vi "LVJSON to Variant.vi"(8 "error in (no error)":errorcluster, 10 "Variant Type":variant, 11 "Root Element in":T1) -> (0 "error out":errorcluster, 2 "Key":string, 3 "Variant out":variant)   [LabVIEW 2019, in "labview_json.lvlib"]
uses:
  labview_json.lvlib
  Element.ctl
  Element Type.ctl
  <vilib>/Utility/error.llb/Error Cluster From Error Code.vi
  <vilib>/ErrorRing/Error Ring.xnode
  <vilib>/Utility/Data Type/NI_Data Type.lvlib
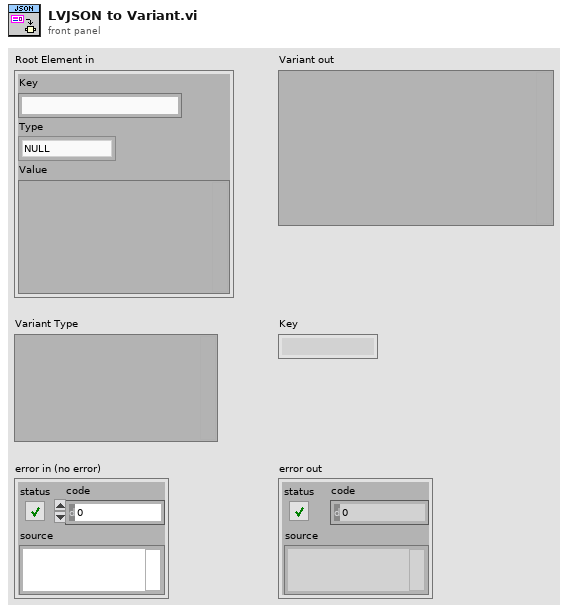
[diagram p1: front panel]
types:
  T1 = typedef "labview_json.lvlib/Element.ctl" = cluster{"Key":string, "Type":T2, "Value":variant}
  T2 = typedef "labview_json.lvlib/Element Type.ctl" = enum8{"NULL", "OBJECT", "ARRAY", "BOOL", "INT", "UINT", "FLOAT", "STRING"}
  T3 = typedef "NI_Data Type.lvlib/Data Type.ctl" = enum8{"Invalid Type", "Void", "I8", "I16", "I32", "I64", "U8", "U16", "U32", "U64", "Single Float", "Double Float", "Extended Float", "Single Complex", "Double Complex", "Extended Complex", "Enum U8", "Enum U16", "Enum U32", "Enum U64", "Single Float With Unit", "Double Float With Unit", "Extended Float With Unit", "Single Complex with Unit", "Double Complex with Unit", "Extended Complex with Unit", "Boolean", "String", "Path", "Picture", "Tag", "Array", "Cluster", "Variant", "LV Variant", "Waveform", "Timestamp", "Digital Waveform", "Digital Data", "ExpressData", "Refnum", "External Data", "VI", "Poly VI", "LabVIEW Class Instance", "Fixed Point", "Set Collection", "Map Collection"}
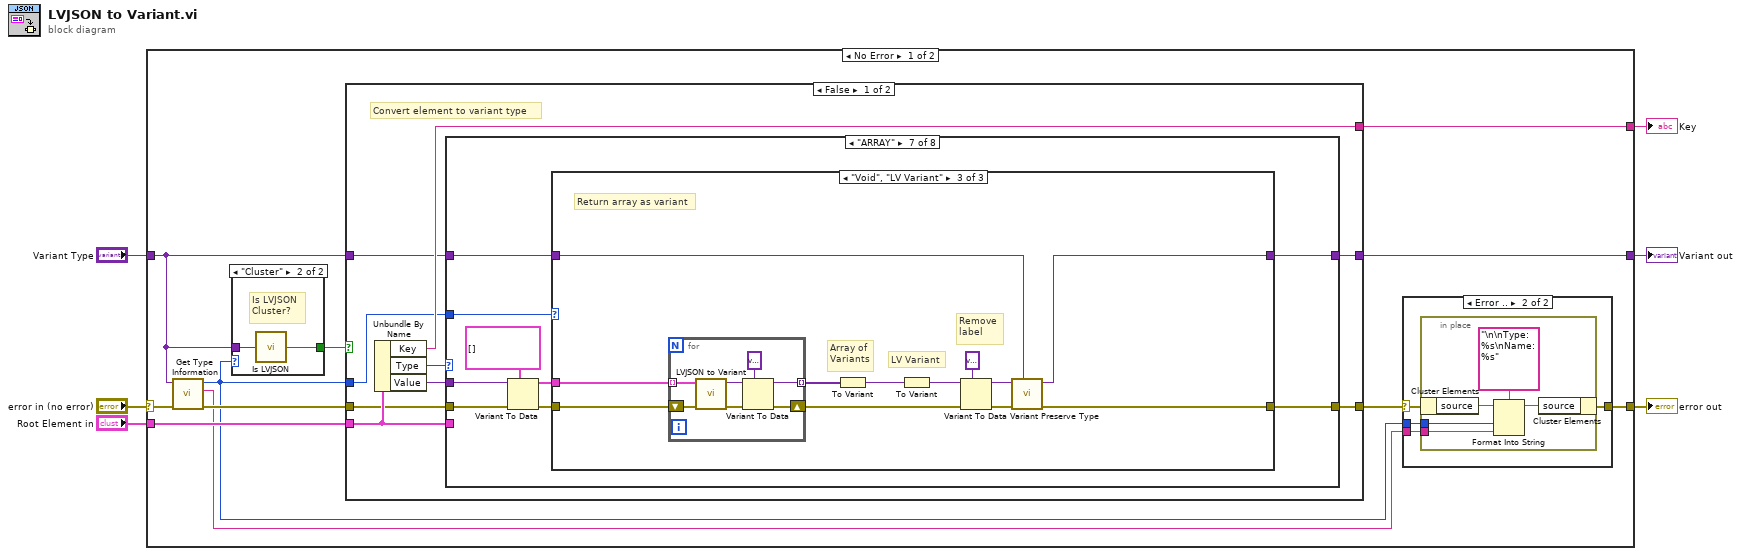
[diagram p0: block diagram]
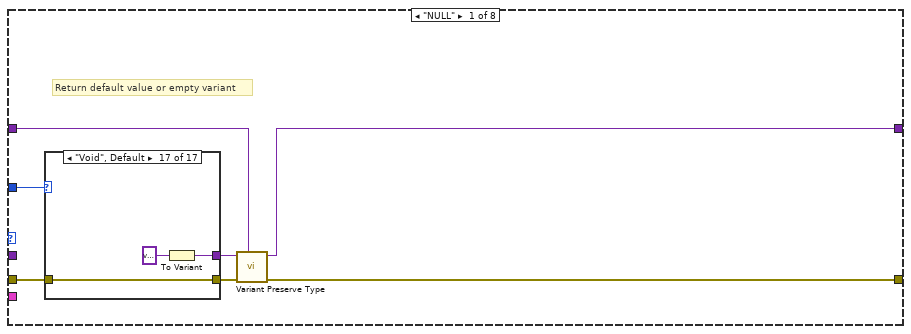
[diagram p2: hidden frame]
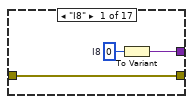
[diagram p3: hidden frame]
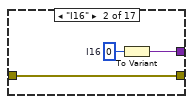
[diagram p4: hidden frame]
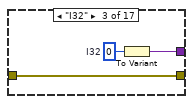
[diagram p5: hidden frame]
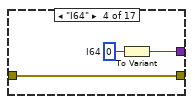
[diagram p6: hidden frame]
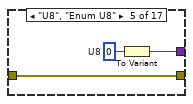
[diagram p7: hidden frame]
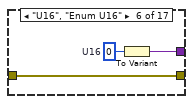
[diagram p8: hidden frame]
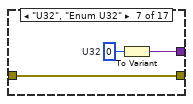
[diagram p9: hidden frame]
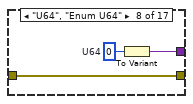
[diagram p10: hidden frame]
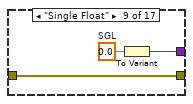
[diagram p11: hidden frame]
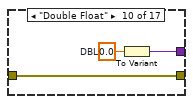
[diagram p12: hidden frame]
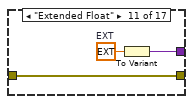
[diagram p13: hidden frame]
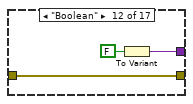
[diagram p14: hidden frame]
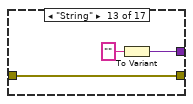
[diagram p15: hidden frame]
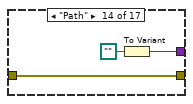
[diagram p16: hidden frame]
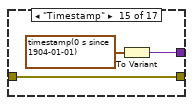
[diagram p17: hidden frame]
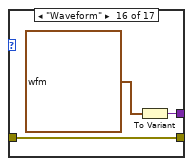
[diagram p18: hidden frame]
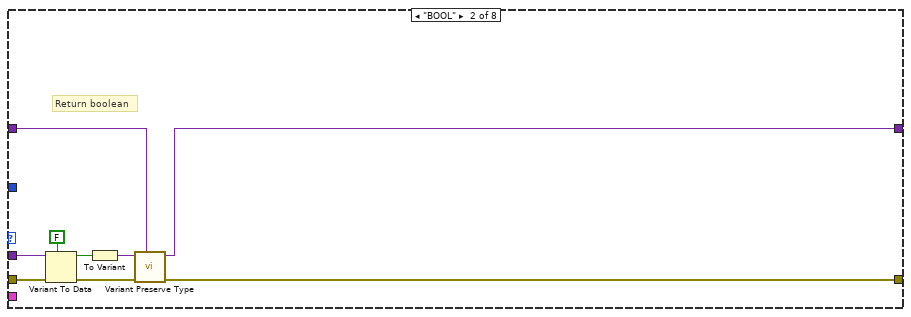
[diagram p19: hidden frame]
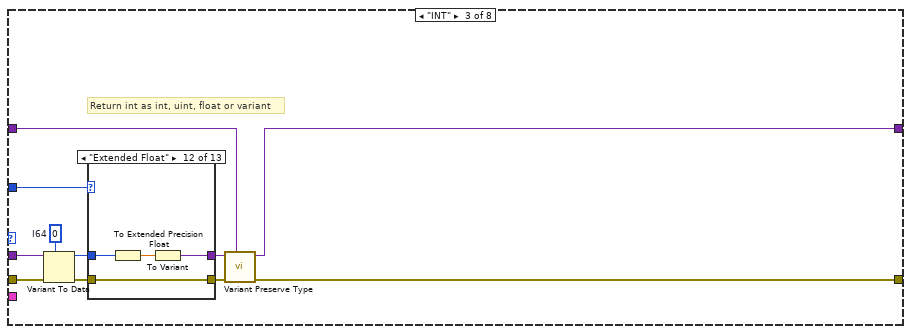
[diagram p20: hidden frame]
diagram:
  n1 = case shown="No Error" "error in (no error)" {
    selector: "error in (no error)" -> [w14 w587]
    tunnel: "Root Element in" -> [w15 _]
    tunnel: [w17 w587] -> w6
    tunnel: "Variant Type" -> [w13 w586]
    tunnel: [w16 _] -> w2
    tunnel: [w12 w586] -> w1
    frame No Error {
      n2 = call <vilib>:"Get Type Information.vi"("error in (no error)"=w14, "variant"=w13) -> ("error out"=w11:errorcluster, "name"=w9:string, "type"=w8:T3)  [unwired: 5 in, 2 out]
      n3 = case shown="\"Cluster\"" w8 {
        tunnel: w13 -> [_ w575]
        tunnel: [_ w574] -> w7
        frame Default {
        }
        frame "Cluster" {
          # "Is LVJSON\nCluster?"
          n4 = call "Is LVJSON.vi"("Variant"=w575) -> ("Is LVJSON?"=w574:bool)
        }
      }
      n5 = case shown="False" w7 {
        tunnel: [w26 w571] -> w16
        tunnel: w15 -> [w25 w572]
        tunnel: w13 -> [w24 _]
        tunnel: [w23 w573] -> w12
        tunnel: w11 -> [w22 w570]
        tunnel: [w21 w570] -> w10
        tunnel: w8 -> [w18 _]
        frame False {
          # "Convert element to variant type"
          n6 = Unbundle By Name(w25) -> ("Key"=w26:string, "Type"=w20:T2, "Value"=w19:variant)
          n7 = case shown="\"ARRAY\"" w20 {
            tunnel: [w31 w93 w104 w166 w228 w290 w343 w434] -> w23
            tunnel: w22 -> [w33 w88 w98 w160 w222 w285 w349 w440]
            tunnel: w24 -> [w29 w91 w102 w164 w226 w282 w344 w435]
            tunnel: w25 -> [_ _ _ _ _ _ _ w432]
            tunnel: w19 -> [_ w87 w97 w159 w221 w284 w348 w439]
            tunnel: w18 -> [w32 _ w96 w156 w220 w283 w347 w438]
            tunnel: [w30 w92 w103 w165 w227 w289 w342 w433] -> w21
            frame "NULL" {
              # "Return default value or empty variant"
              n8 = case shown="\"Void\", Default" w32 {
                tunnel: [w36 w39 w42 w45 w48 w51 w54 w57 w60 w63 w66 w69 w72 w75 w78 w81 w84] -> w28
                tunnel: w33 -> [w36 w39 w42 w45 w48 w51 w54 w57 w60 w63 w66 w69 w72 w75 w78 w81 w84]
                tunnel: [w35 w38 w41 w44 w47 w50 w53 w56 w59 w62 w65 w68 w71 w74 w77 w80 w83] -> w27
                frame "I8" {
                  w34 = i8 0  # I8
                  n9 = To Variant(anything=w34) -> (Variant=w35:variant)
                }
                frame "I16" {
                  w37 = i16 0  # I16
                  n10 = To Variant(anything=w37) -> (Variant=w38:variant)
                }
                frame "I32" {
                  w40 = 0  # I32
                  n11 = To Variant(anything=w40) -> (Variant=w41:variant)
                }
                frame "I64" {
                  w43 = i64 0  # I64
                  n12 = To Variant(anything=w43) -> (Variant=w44:variant)
                }
                frame "U8", "Enum U8" {
                  w46 = u8 0  # U8
                  n13 = To Variant(anything=w46) -> (Variant=w47:variant)
                }
                frame "U16", "Enum U16" {
                  w49 = u16 0  # U16
                  n14 = To Variant(anything=w49) -> (Variant=w50:variant)
                }
                frame "U32", "Enum U32" {
                  w52 = u32 0  # U32
                  n15 = To Variant(anything=w52) -> (Variant=w53:variant)
                }
                frame "U64", "Enum U64" {
                  w55 = u64 0  # U64
                  n16 = To Variant(anything=w55) -> (Variant=w56:variant)
                }
                frame "Single Float" {
                  w58 = sgl 0.0  # SGL
                  n17 = To Variant(anything=w58) -> (Variant=w59:variant)
                }
                frame "Double Float" {
                  w61 = 0.0  # DBL
                  n18 = To Variant(anything=w61) -> (Variant=w62:variant)
                }
                frame "Extended Float" {
                  w64 = ext 0.0  # EXT
                  n19 = To Variant(anything=w64) -> (Variant=w65:variant)
                }
                frame "Boolean" {
                  n20 = To Variant(anything=FALSE) -> (Variant=w68:variant)
                }
                frame "String" {
                  n21 = To Variant(anything="") -> (Variant=w71:variant)
                }
                frame "Path" {
                  n22 = To Variant(anything=path "" ("Not A Path Constant")) -> (Variant=w74:variant)
                }
                frame "Timestamp" {
                  n23 = To Variant(anything=timestamp(0 s since 1904-01-01)) -> (Variant=w77:variant)
                }
                frame "Waveform" {
                  n24 = To Variant(anything=waveform(dbl) {"t0"=timestamp(0 s since 1904-01-01), "dt"=1.0, "Y"=[]} ("Waveform")) -> (Variant=w80:variant)
                }
                frame "Void", Default {
                  n25 = To Variant(anything=variant) -> (Variant=w83:variant)
                }
              }
              n26 = call "Variant Preserve Type.vi"("Variant Type"=w29, "error in (no error)"=w28, "Variant in"=w27) -> ("error out"=w30:errorcluster, "Variant out"=w31:variant)  [unwired: 7 in]
            }
            frame "BOOL" {
              # "Return boolean"
              n27 = Variant To Data(error in=w88, type=FALSE, Variant=w87) -> (data=w90:bool, error out=w86:errorcluster)
              n28 = To Variant(anything=w90) -> (Variant=w85:variant)
              n29 = call "Variant Preserve Type.vi"("Variant Type"=w91, "error in (no error)"=w86, "Variant in"=w85) -> ("error out"=w92:errorcluster, "Variant out"=w93:variant)  [unwired: 7 in]
            }
            frame "INT" {
              w101 = i64 0  # I64
              # "Return int as int, uint, float or variant"
              n30 = Variant To Data(error in=w98, type=w101, Variant=w97) -> (data=w99:i64, error out=w100:errorcluster)
              n31 = case shown="\"Extended Float\"" w96 {
                tunnel: [w107 w110 w114 w118 w122 w126 w130 w134 w138 w142 w146 w150 w155] -> w95
                tunnel: w100 -> [w107 w110 w114 w118 w122 w126 w130 w134 w138 w142 w146 w150 w155]
                tunnel: [w105 w108 w112 w116 w120 w124 w128 w132 w136 w140 w144 w148 w153] -> w94
                tunnel: w99 -> [w106 w111 w115 w119 w123 w127 w131 w135 w139 w143 w147 w151 w154]
                frame "Void", Default {
                  n32 = To Variant(anything=w106) -> (Variant=w105:variant)
                }
                frame "I8" {
                  n33 = To Byte Integer(number=w111) -> (8bit integer=w109:i8)
                  n34 = To Variant(anything=w109) -> (Variant=w108:variant)
                }
                frame "I16" {
                  n35 = To Word Integer(number=w115) -> (16bit integer=w113:i16)
                  n36 = To Variant(anything=w113) -> (Variant=w112:variant)
                }
                frame "I32" {
                  n37 = To Long Integer(number=w119) -> (32bit integer=w117:i32)
                  n38 = To Variant(anything=w117) -> (Variant=w116:variant)
                }
                frame "I64" {
                  n39 = To Quad Integer(1:w123) -> (0:w121:i64)
                  n40 = To Variant(anything=w121) -> (Variant=w120:variant)
                }
                frame "U8", "Enum U8" {
                  n41 = To Unsigned Byte Integer(number=w127) -> (unsigned 8bit integer=w125:u8)
                  n42 = To Variant(anything=w125) -> (Variant=w124:variant)
                }
                frame "U16", "Enum U16" {
                  n43 = To Unsigned Word Integer(number=w131) -> (unsigned 16bit integer=w129:u16)
                  n44 = To Variant(anything=w129) -> (Variant=w128:variant)
                }
                frame "U32", "Enum U32" {
                  n45 = To Unsigned Long Integer(number=w135) -> (unsigned 32bit integer=w133:u32)
                  n46 = To Variant(anything=w133) -> (Variant=w132:variant)
                }
                frame "U64", "Enum U64" {
                  n47 = To Unsigned Quad Integer(1:w139) -> (0:w137:u64)
                  n48 = To Variant(anything=w137) -> (Variant=w136:variant)
                }
                frame "Single Float" {
                  n49 = To Single Precision Float(number=w143) -> (single precision float=w141:sgl)
                  n50 = To Variant(anything=w141) -> (Variant=w140:variant)
                }
                frame "Double Float" {
                  n51 = To Double Precision Float(number=w147) -> (double precision float=w145:dbl)
                  n52 = To Variant(anything=w145) -> (Variant=w144:variant)
                }
                frame "Extended Float" {
                  n53 = To Extended Precision Float(1:w151) -> (0:w149:ext)
                  n54 = To Variant(anything=w149) -> (Variant=w148:variant)
                }
                frame "LV Variant" {
                  n55 = To Variant(anything=w154) -> (Variant=w152:variant)
                  n56 = To Variant(anything=w152) -> (Variant=w153:variant)
                }
              }
              n57 = call "Variant Preserve Type.vi"("Variant Type"=w102, "error in (no error)"=w95, "Variant in"=w94) -> ("error out"=w103:errorcluster, "Variant out"=w104:variant)  [unwired: 7 in]
            }
            frame "UINT" {
              w163 = u64 0  # U64
              # "Return uint as int, uint, float, enum or variant"
              n58 = Variant To Data(error in=w160, type=w163, Variant=w159) -> (data=w161:u64, error out=w162:errorcluster)
              n59 = case shown="\"Extended Float\"" w156 {
                tunnel: [w169 w172 w176 w180 w184 w188 w192 w196 w200 w204 w208 w212 w217] -> w158
                tunnel: w162 -> [w169 w172 w176 w180 w184 w188 w192 w196 w200 w204 w208 w212 w217]
                tunnel: [w167 w170 w174 w178 w182 w186 w190 w194 w198 w202 w206 w210 w215] -> w157
                tunnel: w161 -> [w168 w173 w177 w181 w185 w189 w193 w197 w201 w205 w209 w213 w216]
                frame "Void", Default {
                  n60 = To Variant(anything=w168) -> (Variant=w167:variant)
                }
                frame "I8" {
                  n61 = To Byte Integer(number=w173) -> (8bit integer=w171:i8)
                  n62 = To Variant(anything=w171) -> (Variant=w170:variant)
                }
                frame "I16" {
                  n63 = To Word Integer(number=w177) -> (16bit integer=w175:i16)
                  n64 = To Variant(anything=w175) -> (Variant=w174:variant)
                }
                frame "I32" {
                  n65 = To Long Integer(number=w181) -> (32bit integer=w179:i32)
                  n66 = To Variant(anything=w179) -> (Variant=w178:variant)
                }
                frame "I64" {
                  n67 = To Quad Integer(1:w185) -> (0:w183:i64)
                  n68 = To Variant(anything=w183) -> (Variant=w182:variant)
                }
                frame "U8", "Enum U8" {
                  n69 = To Unsigned Byte Integer(number=w189) -> (unsigned 8bit integer=w187:u8)
                  n70 = To Variant(anything=w187) -> (Variant=w186:variant)
                }
                frame "U16", "Enum U16" {
                  n71 = To Unsigned Word Integer(number=w193) -> (unsigned 16bit integer=w191:u16)
                  n72 = To Variant(anything=w191) -> (Variant=w190:variant)
                }
                frame "U32", "Enum U32" {
                  n73 = To Unsigned Long Integer(number=w197) -> (unsigned 32bit integer=w195:u32)
                  n74 = To Variant(anything=w195) -> (Variant=w194:variant)
                }
                frame "U64", "Enum U64" {
                  n75 = To Unsigned Quad Integer(1:w201) -> (0:w199:u64)
                  n76 = To Variant(anything=w199) -> (Variant=w198:variant)
                }
                frame "Single Float" {
                  n77 = To Single Precision Float(number=w205) -> (single precision float=w203:sgl)
                  n78 = To Variant(anything=w203) -> (Variant=w202:variant)
                }
                frame "Double Float" {
                  n79 = To Double Precision Float(number=w209) -> (double precision float=w207:dbl)
                  n80 = To Variant(anything=w207) -> (Variant=w206:variant)
                }
                frame "Extended Float" {
                  n81 = To Extended Precision Float(1:w213) -> (0:w211:ext)
                  n82 = To Variant(anything=w211) -> (Variant=w210:variant)
                }
                frame "LV Variant" {
                  n83 = To Variant(anything=w216) -> (Variant=w214:variant)
                  n84 = To Variant(anything=w214) -> (Variant=w215:variant)
                }
              }
              n85 = call "Variant Preserve Type.vi"("Variant Type"=w164, "error in (no error)"=w158, "Variant in"=w157) -> ("error out"=w165:errorcluster, "Variant out"=w166:variant)  [unwired: 7 in]
            }
            frame "FLOAT" {
              w225 = 0.0  # DBL
              # "Return float as int, uint, float or variant"
              n86 = Variant To Data(error in=w222, type=w225, Variant=w221) -> (data=w223:dbl, error out=w224:errorcluster)
              n87 = case shown="\"Extended Float\"" w220 {
                tunnel: [w231 w234 w238 w242 w246 w250 w254 w258 w262 w266 w270 w274 w279] -> w218
                tunnel: w224 -> [w231 w234 w238 w242 w246 w250 w254 w258 w262 w266 w270 w274 w279]
                tunnel: [w229 w232 w236 w240 w244 w248 w252 w256 w260 w264 w268 w272 w277] -> w219
                tunnel: w223 -> [w230 w235 w239 w243 w247 w251 w255 w259 w263 w267 w271 w275 w278]
                frame "Void", Default {
                  n88 = To Variant(anything=w230) -> (Variant=w229:variant)
                }
                frame "I8" {
                  n89 = To Byte Integer(number=w235) -> (8bit integer=w233:i8)
                  n90 = To Variant(anything=w233) -> (Variant=w232:variant)
                }
                frame "I16" {
                  n91 = To Word Integer(number=w239) -> (16bit integer=w237:i16)
                  n92 = To Variant(anything=w237) -> (Variant=w236:variant)
                }
                frame "I32" {
                  n93 = To Long Integer(number=w243) -> (32bit integer=w241:i32)
                  n94 = To Variant(anything=w241) -> (Variant=w240:variant)
                }
                frame "I64" {
                  n95 = To Quad Integer(1:w247) -> (0:w245:i64)
                  n96 = To Variant(anything=w245) -> (Variant=w244:variant)
                }
                frame "U8", "Enum U8" {
                  n97 = To Unsigned Byte Integer(number=w251) -> (unsigned 8bit integer=w249:u8)
                  n98 = To Variant(anything=w249) -> (Variant=w248:variant)
                }
                frame "U16", "Enum U16" {
                  n99 = To Unsigned Word Integer(number=w255) -> (unsigned 16bit integer=w253:u16)
                  n100 = To Variant(anything=w253) -> (Variant=w252:variant)
                }
                frame "U32", "Enum U32" {
                  n101 = To Unsigned Long Integer(number=w259) -> (unsigned 32bit integer=w257:u32)
                  n102 = To Variant(anything=w257) -> (Variant=w256:variant)
                }
                frame "U64", "Enum U64" {
                  n103 = To Unsigned Quad Integer(1:w263) -> (0:w261:u64)
                  n104 = To Variant(anything=w261) -> (Variant=w260:variant)
                }
                frame "Single Float" {
                  n105 = To Single Precision Float(number=w267) -> (single precision float=w265:sgl)
                  n106 = To Variant(anything=w265) -> (Variant=w264:variant)
                }
                frame "Double Float" {
                  n107 = To Double Precision Float(number=w271) -> (double precision float=w269:dbl)
                  n108 = To Variant(anything=w269) -> (Variant=w268:variant)
                }
                frame "Extended Float" {
                  n109 = To Extended Precision Float(1:w275) -> (0:w273:ext)
                  n110 = To Variant(anything=w273) -> (Variant=w272:variant)
                }
                frame "LV Variant" {
                  n111 = To Variant(anything=w278) -> (Variant=w276:variant)
                  n112 = To Variant(anything=w276) -> (Variant=w277:variant)
                }
              }
              n113 = call "Variant Preserve Type.vi"("Variant Type"=w226, "error in (no error)"=w218, "Variant in"=w219) -> ("error out"=w227:errorcluster, "Variant out"=w228:variant)  [unwired: 7 in]
            }
            frame "STRING" {
              # "Return string as string, enum, path, timestamp or variant"
              n114 = Variant To Data(error in=w285, type="", Variant=w284) -> (data=w287:string, error out=w288:errorcluster)
              n115 = case shown="\"LV Variant\"" w283 {
                tunnel: [w293 w295 w306 w317 w329 w333 w337 w341] -> w280
                tunnel: w288 -> [w293 w294 w305 w316 w329 w333 w337 w341]
                tunnel: [w291 w304 w315 w326 w328 w332 w335 w340] -> w281
                tunnel: w287 -> [w292 w301 w312 w323 w327 w331 w336 w339]
                tunnel: w282 -> [_ w303 w314 w325 _ _ _ _]
                frame "Void", Default {
                  n116 = To Variant(anything=w292) -> (Variant=w291:variant)
                }
                frame "Enum U8" {
                  n117 = call <vilib>:"Get Numeric Information.vi"("error in (no error)"=w294, "variant"=w303) -> ("error out"=w295:errorcluster, "enum names"=w300:string[])  [unwired: 6 in, 2 out]
                  n118 = Search 1D Array(1D array=w300, element=w301) -> (index of element=w298:i32)  [unwired: 1 in]
                  n119 = Less Than 0?(x=w298) -> (x < 0?=w299:bool)
                  n120 = Select(t=0, s=w299, f=w298) -> (s? t:f=w296:i32)
                  n121 = To Unsigned Byte Integer(number=w296) -> (unsigned 8bit integer=w302:u8)
                  n122 = To Variant(anything=w302) -> (Variant=w304:variant)
                }
                frame "Enum U16" {
                  n123 = call <vilib>:"Get Numeric Information.vi"("error in (no error)"=w305, "variant"=w314) -> ("error out"=w306:errorcluster, "enum names"=w311:string[])  [unwired: 6 in, 2 out]
                  n124 = Search 1D Array(1D array=w311, element=w312) -> (index of element=w309:i32)  [unwired: 1 in]
                  n125 = Less Than 0?(x=w309) -> (x < 0?=w310:bool)
                  n126 = Select(t=0, s=w310, f=w309) -> (s? t:f=w307:i32)
                  n127 = To Unsigned Word Integer(number=w307) -> (unsigned 16bit integer=w313:u16)
                  n128 = To Variant(anything=w313) -> (Variant=w315:variant)
                }
                frame "Enum U32" {
                  n129 = call <vilib>:"Get Numeric Information.vi"("error in (no error)"=w316, "variant"=w325) -> ("error out"=w317:errorcluster, "enum names"=w322:string[])  [unwired: 6 in, 2 out]
                  n130 = Search 1D Array(1D array=w322, element=w323) -> (index of element=w320:i32)  [unwired: 1 in]
                  n131 = Less Than 0?(x=w320) -> (x < 0?=w321:bool)
                  n132 = Select(t=0, s=w321, f=w320) -> (s? t:f=w318:i32)
                  n133 = To Unsigned Long Integer(number=w318) -> (unsigned 32bit integer=w324:u32)
                  n134 = To Variant(anything=w324) -> (Variant=w326:variant)
                }
                frame "String" {
                  n135 = To Variant(anything=w327) -> (Variant=w328:variant)
                }
                frame "Path" {
                  n136 = String To Path(string=w331) -> (path=w330:path)
                  n137 = To Variant(anything=w330) -> (Variant=w332:variant)
                }
                frame "LV Variant" {
                  n138 = To Variant(anything=w336) -> (Variant=w334:variant)
                  n139 = To Variant(anything=w334) -> (Variant=w335:variant)
                }
                frame "Timestamp" {
                  n140 = call "JSON ISO8601 to Timestamp.vi"("ISO 8601 Date Time"=w339) -> ("Local Time Stamp"=w338:timestamp)  [unwired: 10 in]
                  n141 = To Variant(anything=w338) -> (Variant=w340:variant)
                }
              }
              n142 = call "Variant Preserve Type.vi"("Variant Type"=w282, "error in (no error)"=w280, "Variant in"=w281) -> ("error out"=w289:errorcluster, "Variant out"=w290:variant)  [unwired: 7 in]
            }
            frame "ARRAY" {
              n143 = Variant To Data(error in=w349, type=T1[] [], Variant=w348) -> (data=w345:T1[], error out=w346:errorcluster)
              n144 = case shown="\"Void\", \"LV Variant\"" w347 {
                tunnel: [w351 w363 w420] -> w342
                tunnel: w346 -> [w352 w366 w422]
                tunnel: w345 -> [_ w362 w424]
                tunnel: w344 -> [w354 w360 w418]
                tunnel: [w354 w359 w419] -> w343
                frame Default {
                  n145 = xnode "Error Ring"() -> ("error out"=w353:errorcluster)
                  n146 = Merge Errors(w352, w353) -> (w351:errorcluster)
                }
                frame "Array" {
                  # "Return array"
                  n147 = call <vilib>:"Get Array Information.vi"("error in (no error)"=w366, "variant"=w360) -> ("error out"=w364:errorcluster, "array element data type"=w361:variant, "number of dimensions"=w365:i32)  [unwired: 6 in, 1 out]
                  n148 = case shown="1" w365 {
                    tunnel: w364 -> [w369 w376]
                    tunnel: [w368 w383] -> w363
                    tunnel: w362 -> [_ w388]
                    tunnel: w361 -> [_ w377]
                    tunnel: [w367 w381] -> w359
                    tunnel: w360 -> [w367 w380]
                    frame Default {
                      n149 = xnode "Error Ring"() -> ("error out"=w370:errorcluster)
                      n150 = Merge Errors(w369, w370) -> (w368:errorcluster)
                    }
                    frame 1 {
                      n151 = Variant To Data(error in=w376, type=variant[] [], Variant=w380) -> (data=w379:variant[], error out=w375:errorcluster)
                      n152 = Array Size(array=w379) -> (size(s)=w378:i32)
                      n153 = call <vilib>:"Get Type Information.vi"("error in (no error)"=w375, "variant"=w377) -> ("error out"=w387:errorcluster, "type"=w385:T3)  [unwired: 5 in, 3 out]
                      n154 = for {
                        tunnel: w388 -> [w411] mode=indexing
                        shift-right: [w410] -> w390
                        shift-left: w387 -> [w412]
                        tunnel: [w409] -> w389 mode=indexing
                        tunnel: w379 -> [w405]
                        tunnel: w378 -> [w403]
                        tunnel: w377 -> [w400]
                        i -> [w404]
                        n155 = Less?(x=w404, y=w403) -> (x < y?=w402:bool)
                        n156 = Index Array(array=w405, index=w404) -> (element=w401:variant)
                        n157 = Select(t=w401, s=w402, f=w400) -> (s? t:f=w399:variant)
                        n158 = call "LVJSON to Variant.vi"("error in (no error)"=w412, "Variant Type"=w399, "Root Element in"=w411) -> ("error out"=w407:errorcluster, "Variant out"=w406:variant)  [unwired: 6 in, 1 out]
                        n159 = Variant To Data(error in=w407, type=variant, Variant=w406) -> (data=w409:variant, error out=w410:errorcluster)
                      }
                      n160 = case shown="Default" w385 {
                        tunnel: w390 -> [w391 w398]
                        tunnel: w389 -> [w393 w397]
                        tunnel: [w392 w396] -> w382
                        tunnel: [w391 w395] -> w384
                        tunnel: w377 -> [_ w394]
                        frame "Void", "LV Variant" {
                          n161 = To Variant(anything=w393) -> (Variant=w392:variant)
                        }
                        frame Default {
                          n162 = call "Variant Create Array.vi"("error in (no error)"=w398, "Default Type (if empty)"=w394, "Elements"=w397) -> ("error out"=w395:errorcluster, "Array"=w396:variant)  [unwired: 7 in]
                        }
                      }
                      n163 = call "Variant Preserve Type.vi"("Variant Type"=w380, "error in (no error)"=w384, "Variant in"=w382) -> ("error out"=w383:errorcluster, "Variant out"=w381:variant)  [unwired: 7 in]
                    }
                  }
                }
                frame "Void", "LV Variant" {
                  # "Remove\nlabel"
                  # "LV Variant"
                  # "Array of\nVariants"
                  # "Return array as variant"
                  n164 = for {
                    tunnel: w424 -> [w430] mode=indexing
                    shift-right: [w426] -> w415
                    shift-left: w422 -> [w431]
                    tunnel: [w425] -> w421 mode=indexing
                    n165 = call "LVJSON to Variant.vi"("error in (no error)"=w431, "Root Element in"=w430) -> ("error out"=w428:errorcluster, "Variant out"=w427:variant)  [unwired: 7 in, 1 out]
                    n166 = Variant To Data(error in=w428, type=variant, Variant=w427) -> (data=w425:variant, error out=w426:errorcluster)
                  }
                  n167 = To Variant(anything=w421) -> (Variant=w423:variant)
                  n168 = To Variant(anything=w423) -> (Variant=w416:variant)
                  n169 = Variant To Data(error in=w415, type=variant, Variant=w416) -> (data=w413:variant, error out=w414:errorcluster)
                  n170 = call "Variant Preserve Type.vi"("Variant Type"=w418, "error in (no error)"=w414, "Variant in"=w413) -> ("error out"=w420:errorcluster, "Variant out"=w419:variant)  [unwired: 7 in]
                }
              }
            }
            frame "OBJECT" {
              n171 = Variant To Data(error in=w440, type=T1[] [], Variant=w439) -> (data=w436:T1[], error out=w437:errorcluster)
              n172 = case shown="\"Cluster\"" w438 {
                tunnel: [w442 w463 w522 w524 w548] -> w433
                tunnel: w437 -> [w443 w459 w504 w526 w550]
                tunnel: w436 -> [_ w458 _ w525 w549]
                tunnel: w435 -> [w445 w460 w503 _ _]
                tunnel: [w445 w462 w521 w523 w546] -> w434
                tunnel: w432 -> [_ _ w500 _ _]
                frame Default {
                  n173 = xnode "Error Ring"() -> ("error out"=w444:errorcluster)
                  n174 = Merge Errors(w443, w444) -> (w442:errorcluster)
                }
                frame "Cluster" {
                  # "Return cluster"
                  n175 = Variant To Data(error in=w459, type=variant[] [], Variant=w460) -> (data=w454:variant[], error out=w457:errorcluster)
                  n176 = Array Size(array=w454) -> (size(s)=w456:i32)
                  n177 = Index Array(array=w454) -> (element=w453:variant)  [unwired: 1 in]
                  n178 = Equal?(x=w456, y=1) -> (x = y?=w451:bool)
                  n179 = Empty String/Path?(string/path=w453) -> (empty?=w452:bool)
                  n180 = And(x=w451, y=w452) -> (x .and. y?=w450:bool)
                  n181 = case shown="False" w450 {
                    tunnel: [w474 w498] -> w463
                    tunnel: [w473 w499] -> w462
                    tunnel: w460 -> [w472 w499]
                    tunnel: w458 -> [w471 _]
                    tunnel: w457 -> [w470 w498]
                    tunnel: w456 -> [w465 _]
                    tunnel: w454 -> [w464 _]
                    frame False {
                      n182 = for {
                        N: w465 -> [_]
                        shift-right: [w475] -> w469
                        shift-left: w470 -> [w476]
                        shift-right: [w478] -> w467
                        shift-left: w464 -> [w480]
                        tunnel: w471 -> [w477]
                        i -> [w479]
                        n183 = in-place {
                          in-place-border: w477 -> [w482]
                          n184 = in-place-array #1(w480, w479) -> (w490:variant)
                          n185 = in-place-match #2(w476) -> (w487:errorcluster)
                          n186 = call <vilib>:"Get Type Information.vi"("error in (no error)"=w487, "variant"=w490) -> ("error out"=w486:errorcluster, "name"=w485:string)  [unwired: 5 in, 3 out]
                          n187 = call "LVJSON Find.vi"("Key"=w485, "Elements in"=w482) -> ("Found?"=w484:bool, "Index"=w483:i32)  [unwired: 8 in]
                          n188 = Index Array(array=w482, index=w483) -> (element=w481:T1)
                          n189 = case shown="True" w484 {
                            tunnel: w490 -> [w492 w493]
                            tunnel: [w492 w497] -> w489
                            tunnel: [w491 w496] -> w488
                            tunnel: w486 -> [w491 w495]
                            tunnel: w481 -> [_ w494]
                            frame False {
                              # "Key not\nfound,\nreturn type"
                            }
                            frame True {
                              # "Key\nFound"
                              n190 = call "LVJSON to Variant.vi"("error in (no error)"=w495, "Variant Type"=w493, "Root Element in"=w494) -> ("error out"=w496:errorcluster, "Variant out"=w497:variant)  [unwired: 6 in, 1 out]
                            }
                          }
                          n191 = in-place-array #1(w489) -> (w478:variant[])  [unwired: 1 out]
                          n192 = in-place-match #2(w488) -> (w475:errorcluster)
                        }
                      }
                      n193 = call "Variant Create Cluster.vi"("error in (no error)"=w469, "Elements"=w467) -> ("error out"=w468:errorcluster, "Cluster"=w466:variant)  [unwired: 8 in]
                      n194 = call "Variant Preserve Type.vi"("Variant Type"=w472, "error in (no error)"=w468, "Variant in"=w466) -> ("error out"=w474:errorcluster, "Variant out"=w473:variant)  [unwired: 7 in]
                    }
                    frame True {
                    }
                  }
                }
                frame "Waveform" {
                  # "Return object as analog waveform"
                  n195 = Variant To Data(error in=w504, type=waveform(dbl) {"t0"=timestamp(0 s since 1904-01-01), "dt"=1.0, "Y"=[]} ("Waveform"), Variant=w503) -> (data=w514:waveform(dbl), error out=w505:errorcluster)
                  n196 = Unbundle By Name(w514) -> ("t0"=w520:timestamp, "dt"=w519:dbl, "Y"=w518:dbl[])
                  n197 = Bundle By Name(cluster=cluster{"t0":timestamp, "dt":dbl, "Y":dbl[]} {"t0"=timestamp(0 s since 1904-01-01), "dt"=0.0, "Y"=[]} ("Waveform"), "t0"=w520, "dt"=w519, "Y"=w518) -> (w515:cluster{"t0":timestamp, "dt":dbl, "Y":dbl[]})
                  n198 = To Variant(anything=w515) -> (Variant=w508:variant)
                  n199 = call "LVJSON to Variant.vi"("error in (no error)"=w505, "Variant Type"=w508, "Root Element in"=w500) -> ("error out"=w517:errorcluster, "Variant out"=w516:variant)  [unwired: 6 in, 1 out]
                  n200 = Variant To Data(error in=w517, type=w515, Variant=w516) -> (data=w513:cluster{"t0":timestamp, "dt":dbl, "Y":dbl[]}, error out=w502:errorcluster)
                  n201 = Unbundle By Name(w513) -> ("t0"=w510:timestamp, "dt"=w511:dbl, "Y"=w512:dbl[])
                  n202 = Bundle By Name(cluster=w514, "t0"=w510, "dt"=w511, "Y"=w512) -> (w509:waveform(dbl))
                  n203 = To Variant(anything=w509) -> (Variant=w501:variant)
                  n204 = call "Variant Preserve Type.vi"("Variant Type"=w503, "error in (no error)"=w502, "Variant in"=w501) -> ("error out"=w522:errorcluster, "Variant out"=w521:variant)  [unwired: 7 in]
                }
                frame "Void" {
                  # "Return object as cluster variant"
                  n205 = for {
                    tunnel: w525 -> [w544] mode=indexing
                    shift-right: [w542] -> w530
                    shift-left: w526 -> [w545]
                    tunnel: [w543] -> w531 mode=indexing
                    tunnel: [w541] -> w529 mode=indexing
                    n206 = call "LVJSON to Variant.vi"("error in (no error)"=w545, "Root Element in"=w544) -> ("error out"=w542:errorcluster, "Key"=w541:string, "Variant out"=w543:variant)  [unwired: 7 in]
                  }
                  n207 = for {
                    tunnel: w531 -> [w538] mode=indexing
                    tunnel: w529 -> [w539] mode=indexing
                    shift-right: [w534] -> w528
                    shift-left: w530 -> [w540]
                    tunnel: [w532] -> w527 mode=indexing
                    # "Set cluster element names"
                    n208 = call <vilib>:"Set Type Information.vi"("error in (no error)"=w540, "Name"=w539, "Variant in"=w538) -> ("error out"=w535:errorcluster, "Variant out"=w537:variant)  [unwired: 7 in]
                    n209 = Variant To Flattened String(Variant=w538) -> (data string=w533:string)  [unwired: 1 out]
                    n210 = Variant To Flattened String(Variant=w537) -> (1:w536:i16[])  [unwired: 1 out]
                    n211 = Flattened String To Variant(4:w535, 6:w533, 7:w536) -> (0:w534:errorcluster, 3:w532:variant)
                  }
                  n212 = call "Variant Create Cluster.vi"("error in (no error)"=w528, "Elements"=w527) -> ("error out"=w524:errorcluster, "Cluster"=w523:variant)  [unwired: 8 in]
                }
                frame "LV Variant" {
                  # "Return object as cluster variant"
                  n213 = for {
                    tunnel: w549 -> [w568] mode=indexing
                    shift-right: [w566] -> w554
                    shift-left: w550 -> [w569]
                    tunnel: [w567] -> w555 mode=indexing
                    tunnel: [w565] -> w553 mode=indexing
                    n214 = call "LVJSON to Variant.vi"("error in (no error)"=w569, "Root Element in"=w568) -> ("error out"=w566:errorcluster, "Key"=w565:string, "Variant out"=w567:variant)  [unwired: 7 in]
                  }
                  n215 = for {
                    tunnel: w555 -> [w562] mode=indexing
                    tunnel: w553 -> [w563] mode=indexing
                    shift-right: [w558] -> w552
                    shift-left: w554 -> [w564]
                    tunnel: [w556] -> w551 mode=indexing
                    # "Set cluster element names"
                    n216 = call <vilib>:"Set Type Information.vi"("error in (no error)"=w564, "Name"=w563, "Variant in"=w562) -> ("error out"=w559:errorcluster, "Variant out"=w561:variant)  [unwired: 7 in]
                    n217 = Variant To Flattened String(Variant=w562) -> (data string=w557:string)  [unwired: 1 out]
                    n218 = Variant To Flattened String(Variant=w561) -> (1:w560:i16[])  [unwired: 1 out]
                    n219 = Flattened String To Variant(4:w559, 6:w557, 7:w560) -> (0:w558:errorcluster, 3:w556:variant)
                  }
                  n220 = call "Variant Create Cluster.vi"("error in (no error)"=w552, "Elements"=w551) -> ("error out"=w548:errorcluster, "Cluster"=w547:variant)  [unwired: 8 in]
                  n221 = To Variant(anything=w547) -> (Variant=w546:variant)
                }
              }
            }
          }
        }
        frame True {
          # "Return LVJSON"
          n222 = Unbundle By Name(w572) -> ("Key"=w571:string)
          n223 = To Variant(anything=w572) -> (Variant=w573:variant)
        }
      }
      n224 = case shown="Error .." w10 {
        selector: w10 -> [w576 w580]
        tunnel: [w576 w579] -> w17
        tunnel: w8 -> [_ w578]
        tunnel: w9 -> [_ w577]
        frame No Error {
        }
        frame Error {
          n225 = in-place {
            in-place-border: w578 -> [w582]
            in-place-border: w577 -> [w581]
            n226 = in-place-cluster #3(w580) -> ("source"=w585:string)
            n227 = Format Into String(format string="\n\nType: %s\nName: %s", initial string=w585, w582, w581) -> (resulting string=w584:string)  [unwired: 1 in, 1 out]
            n228 = in-place-cluster #3("source"=w584) -> (w579:errorcluster)
          }
        }
      }
    }
    frame Error {
    }
  }
  "error out" <- w6
  "Variant out" <- w1
  "Key" <- w2
